vi "BasicArray.vi"() -> ()   [LabVIEW 2019]
panel:
  out "Numeric 2":dbl
  in  "Numeric":dbl
  out "4DaInd":dbl[][][][](array[numeric])
  in  "4Da":dbl[][][][](array[numeric])
  out "3DaInd":dbl[][][](array[numeric])
  in  "3Da":dbl[][][](array[numeric])
  out "2DaInd":dbl[][](array[numeric])
  in  "2Da":dbl[][](array[numeric])
  out "aInd":dbl[](array[numeric])
  in  "a":dbl[](array[numeric])
  # "a[4] = {1,2,3,4}"
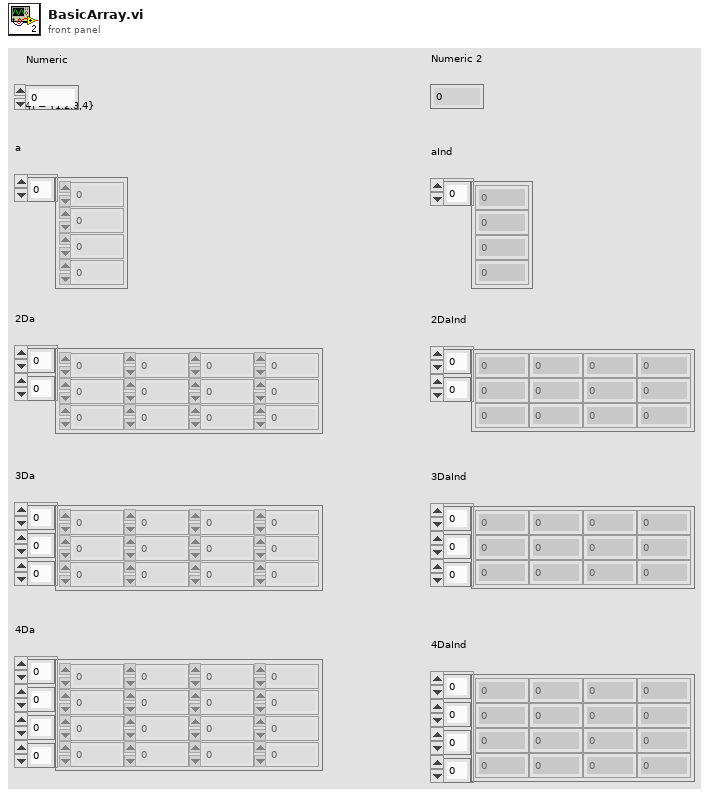
[diagram p1: front panel]
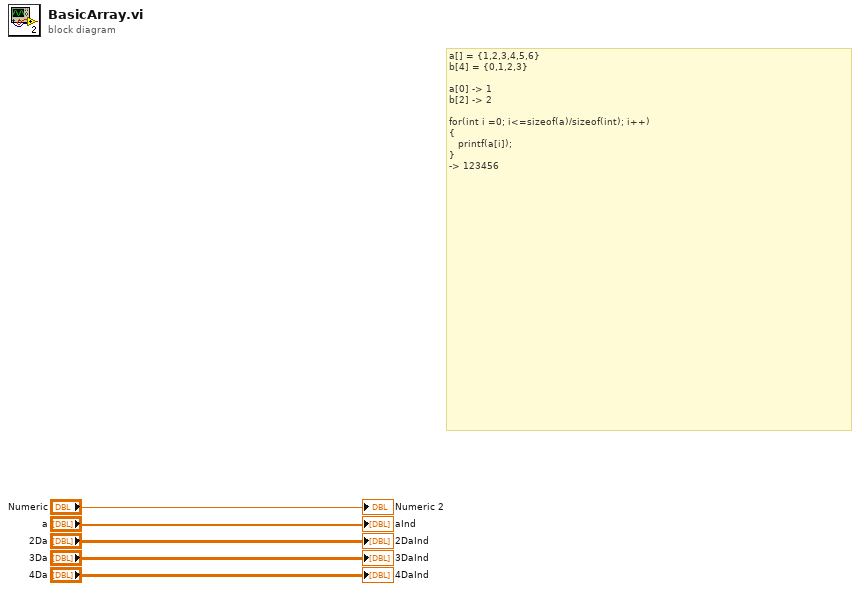
[diagram p0: block diagram]
diagram:
  # "a[] = {1,2,3,4,5,6}\nb[4] = {0,1,2,3}\n\na[0] -> 1\nb[2] -> 2\n\nfor(int i =0; i<=sizeof(a)/sizeof(int); i++)\n{\n   printf(a[i]);\n} \n-> 123456"
  "aInd" <- "a"
  "2DaInd" <- "2Da"
  "3DaInd" <- "3Da"
  "4DaInd" <- "4Da"
  "Numeric 2" <- "Numeric"
